vi "Ex 02 - Simple A-Scan (Low Level).vi"() -> ()   [LabVIEW 2026]
uses:
  <instrlib>/MicroPulse/Public/Data/Datatypes/TCP config.ctl
  <instrlib>/MicroPulse/Public/Data/Datatypes/MP - data output format.ctl
  <instrlib>/MicroPulse/Public/Data/Datatypes/MP - pulser voltage.ctl
  <instrlib>/MicroPulse/Public/Data/Datatypes/MP - pulse damping.ctl
  <instrlib>/MicroPulse/Public/Data/Datatypes/MP - frequency filter.ctl
  <instrlib>/MicroPulse/Public/Data/Datatypes/MP - waveform type.ctl
  <instrlib>/MicroPulse/Public/Data/Datatypes/MP - amplitude reporting mode.ctl
  <instrlib>/MicroPulse/Public/Data/Datatypes/MP - averaging.ctl
  <instrlib>/MicroPulse/Public/Data/Datatypes/MP - echo gate mode.ctl
  <instrlib>/MicroPulse/MicroPulse_Driver.lvlib
  <vilib>/ptbypt/NI_PtbyPt.lvlib
panel:
  out "Test No. Added":u32
  out "num messages":i32
  out "running average PRF":dbl format="%0.2f"
  out "error out":errorcluster
  out "System Messages":string
  out "Waveform Graph":u16[](graph)
  in  "stop":bool
  in  "TCP config":T1={"Connection ID"=refnum, "IP address"="10.1.1.2", "host port"=1067, "OC timeout"=5000, "Read timeout"=100, "Write timeout"=100} {"Write timeout" format="%dms"; "Read timeout" format="%dms"; "OC timeout" format="%dms"}
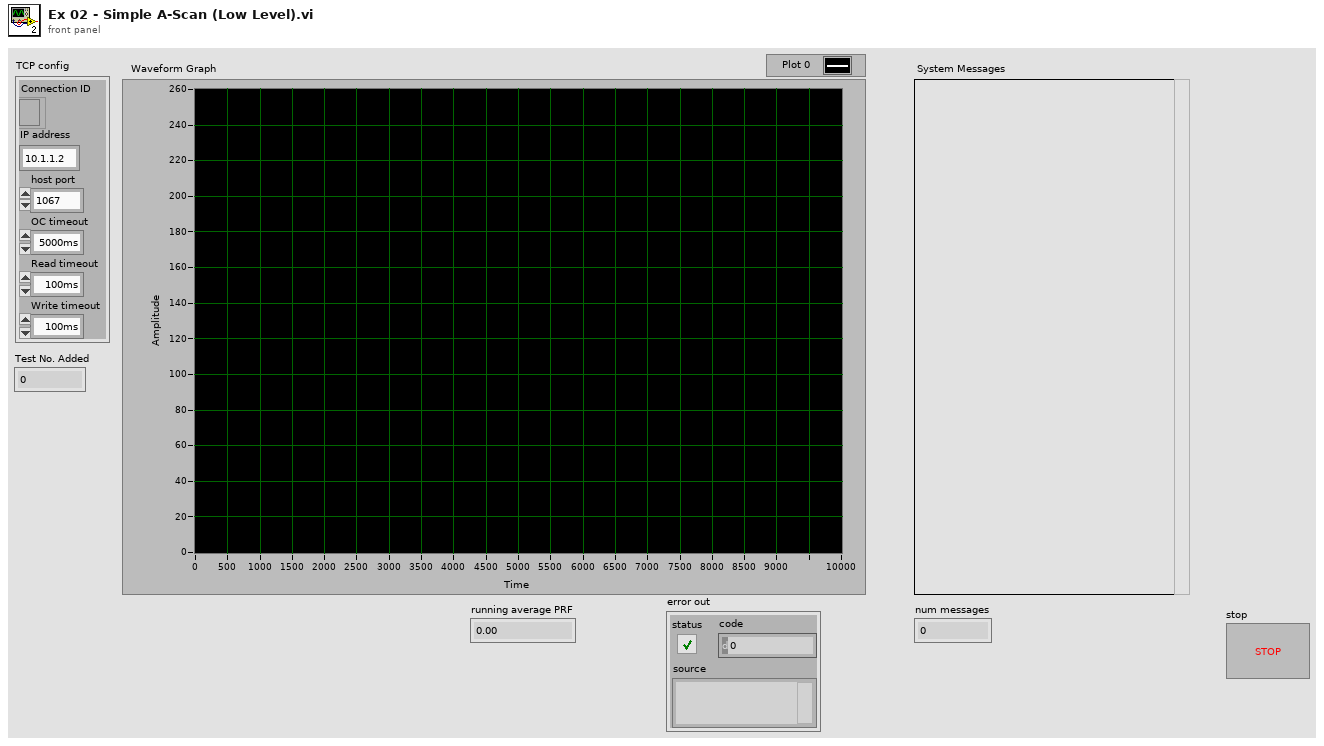
[diagram p1: front panel]
types:
  T1 = typedef "MicroPulse_Driver.lvlib/TCP config.ctl" = cluster{"Connection ID":refnum<k5>, "IP address":string, "host port":u16, "OC timeout":i32, "Read timeout":i32, "Write timeout":i32}
  T2 = typedef "MicroPulse_Driver.lvlib/MP - echo gate mode.ctl" = enum16{"Echo Trigger OFF", "Echo Gate Display Mode", "Echo Trigger ON", "Multi Gate or FMC Mode", "Reserved", "PA - Echo Trigger ON"}
  T3 = typedef "MicroPulse_Driver.lvlib/MP - averaging.ctl" = enum16{"None", "2", "4", "8", "16", "32", "64", "128", "256"}
  T4 = typedef "MicroPulse_Driver.lvlib/MP - amplitude reporting mode.ctl" = enum16{"1st Peak in gate", "Maximum Peak in gate", "All Peaks", "Ascan Data", "1st Threshold Crossing Peak", "Ascan + Peaks", "All Peaks for Multigate", "Peaks + Ascan for Multigate", "Peaks + P_Ascan for Multigate", "Full Matrix Capture"}
  T5 = typedef "MicroPulse_Driver.lvlib/MP - waveform type.ctl" = enum16{"Rectified Signal", "RF Signal", "+Half Wave", "-Half Wave"}
  T6 = typedef "MicroPulse_Driver.lvlib/MP - frequency filter.ctl" = enum16{"No change", "1MHz Bandpass", "2MHz Bandpass", "4MHz Bandpass", "5MHz Bandpass", "10MHz Bandpass", "2.5-18MHz Broadband", "0.75-12MHz  Broadband", "0.5MHz Bandpass", "5MHz 2nd Order TOFD", "10MHz 2nd Order TOFD", "3.0-25MHz Broadband", "3.0-30MHz Broadband"}
  T7 = typedef "MicroPulse_Driver.lvlib/MP - pulse damping.ctl" = enum16{"660W", "458W", "220W", "149W", "102W", "82W", "63W", "51W"}
  T8 = typedef "MicroPulse_Driver.lvlib/MP - pulser voltage.ctl" = enum16{"50V", "100V", "150V", "200V", "250V", "300V"}
  T9 = typedef "MicroPulse_Driver.lvlib/MP - data output format.ctl" = enum16{"", "8-bit Mode", "10-bit Mode", "12-bit Mode", "16-bit Mode", "8-bit Log Mode", "12-bit Packed Mode"}
  T10 = typedef "MicroPulse_Driver.lvlib/MP - scan data info.ctl" = cluster{"Message Header":u16, "Error Message":u16, "Test No.":u32, "Channel No.":u8, "Sweep No.":u32, "Gate No.":u32, "DOF":T9, "retain data":T11, "scan data":u16[], "scan length":i32, "scan index":i32, "peak data":cluster{"timebase":u16[], "data":u16[]}, "#peaks":i32, "PRF":dbl, "IP":cluster{"Axis No.":u8, "Location":u32, "MIP location":u32, "MIP?":bool}, "echo range":u16, "ETG":bool, "CAL 0 complete":bool, "Axis Positions":T12}
  T11 = typedef "MicroPulse_Driver.lvlib/MP - retain scan.ctl" = enum16{"None", "Ascan", "Peaks"}
  T12 = typedef "MicroPulse_Driver.lvlib/MP - axis positions (LLC).ctl" = cluster{"Axis 1":u32, "Axis 2":u32, "Axis 3":u32, "Axis 4":u32, "Status":u8}
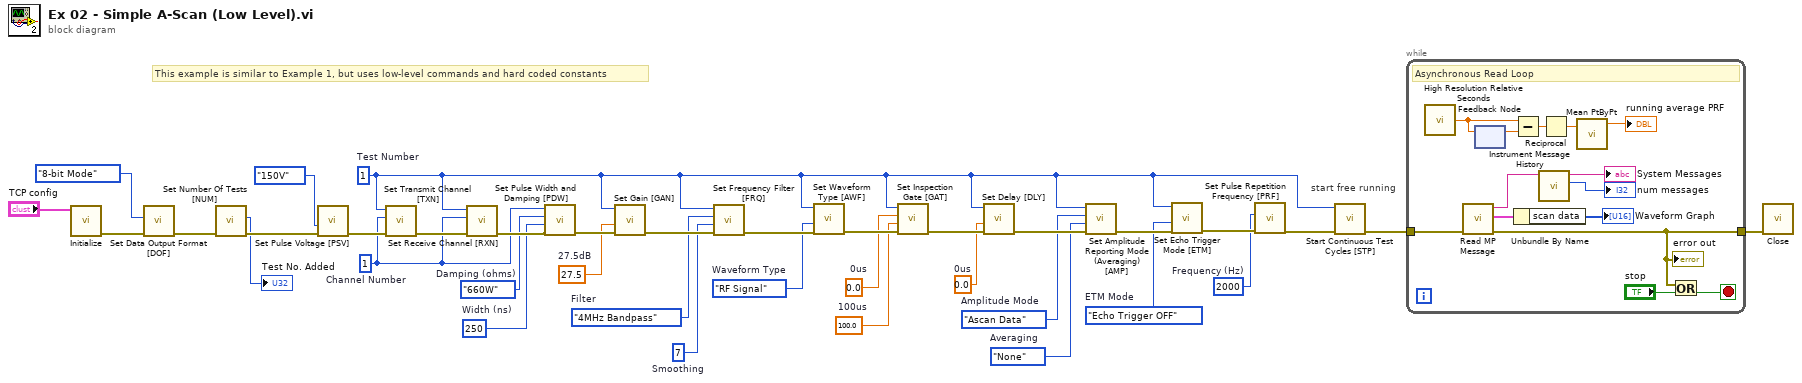
[diagram p0: block diagram]
diagram:
  w9 = u16 2000  # Frequency (Hz)
  w11 = MP_-_echo_gate_mode."Echo Trigger OFF"  # ETM Mode
  w13 = MP_-_averaging."None"  # Averaging
  w14 = MP_-_amplitude_reporting_mode."Ascan Data"  # Amplitude Mode
  w16 = 0.0  # 0us
  w18 = 100.0  # 100us
  w19 = 0.0  # 0us
  w21 = MP_-_waveform_type."RF Signal"  # Waveform Type
  w23 = u16 7  # Smoothing
  w24 = MP_-_frequency_filter."4MHz Bandpass"  # Filter
  w26 = 27.5  # 27.5dB
  w28 = u32 250  # Width (ns)
  w29 = MP_-_pulse_damping."660W"  # Damping (ohms)
  w30 = u32 1  # Channel Number
  w4 = u32 1  # Test Number
  # "This example is similar to Example 1, but uses low-level commands and hard coded constants"
  # "start free running"
  n1 = call <instrlib>:"Initialize.vi"("TCP config"="TCP config") -> ("error out"=w3:errorcluster)  [unwired: 9 in, 1 out]
  n2 = call "Set Data Output Format [DOF].vi"("error in (no error)"=w3, "Mode"=MP_-_data_output_format."8-bit Mode") -> ("error out"=w8:errorcluster)  [unwired: 8 in, 1 out]
  n3 = call <instrlib>:"Set Number Of Tests [NUM].vi"("error in (no error)"=w8) -> ("error out"=w7:errorcluster, "Test No. Added"=→"Test No. Added":u32)  [unwired: 8 in, 1 out]
  n4 = call <instrlib>:"Set Pulse Voltage [PSV].vi"("error in (no error)"=w7, "Voltage"=MP_-_pulser_voltage."150V") -> ("error out"=w33:errorcluster)  [unwired: 8 in, 1 out]
  n5 = call <instrlib>:"Set Transmit Channel [TXN].vi"("error in (no error)"=w33, "Channel Number"=w30, "Test Number"=w4) -> ("error out"=w32:errorcluster)  [unwired: 7 in, 1 out]
  n6 = call <instrlib>:"Set Receive Channel [RXN].vi"("error in (no error)"=w32, "Channel Number"=w30, "Test Number"=w4) -> ("error out"=w31:errorcluster)  [unwired: 7 in, 1 out]
  n7 = call <instrlib>:"Set Pulse Width and Damping [PDW].vi"("error in (no error)"=w31, "Width (ns)"=w28, "Damping"=w29, "Channel Number"=w30) -> ("error out"=w27:errorcluster)  [unwired: 6 in, 1 out]
  n8 = call <instrlib>:"Set Gain [GAN].vi"("error in (no error)"=w27, "Gain (dB)"=w26, "Test Number"=w4) -> ("error out"=w25:errorcluster)  [unwired: 7 in, 1 out]
  n9 = call <instrlib>:"Set Frequency Filter [FRQ].vi"("error in (no error)"=w25, "Smoothing"=w23, "Filter"=w24, "Test Number"=w4) -> ("error out"=w22:errorcluster)  [unwired: 6 in, 1 out]
  n10 = call <instrlib>:"Set Waveform Type [AWF].vi"("error in (no error)"=w22, "Waveform Type"=w21, "Test Number"=w4) -> ("error out"=w20:errorcluster)  [unwired: 7 in, 1 out]
  n11 = call <instrlib>:"Set Inspection Gate [GAT].vi"("error in (no error)"=w20, "Gate Length (us)"=w18, "Gate Start (us)"=w19, "Test Number"=w4) -> ("error out"=w17:errorcluster)  [unwired: 6 in, 1 out]
  n12 = call <instrlib>:"Set Delay [DLY].vi"("error in (no error)"=w17, "Delay (us)"=w16, "Test Number"=w4) -> ("error out"=w15:errorcluster)  [unwired: 7 in, 1 out]
  n13 = call <instrlib>:"Set Amplitude Reporting Mode (Averaging) [AMP].vi"("error in (no error)"=w15, "Averaging"=w13, "Amplitude Mode"=w14, "Test Number"=w4) -> ("error out"=w12:errorcluster)  [unwired: 6 in, 1 out]
  n14 = call <instrlib>:"Set Echo Trigger Mode [ETM].vi"("error in (no error)"=w12, "ETM Mode"=w11, "Test Number"=w4) -> ("error out"=w10:errorcluster)  [unwired: 7 in, 1 out]
  n15 = call <instrlib>:"Set Pulse Repetition Frequency [PRF].vi"("error in (no error)"=w10, "Frequency (Hz)"=w9) -> ("error out"=w6:errorcluster)  [unwired: 8 in, 1 out]
  n16 = call <instrlib>:"Start Continuous Test Cycles [STP].vi"("error in (no error)"=w6, "Test Number"=w4) -> ("error out"=w2:errorcluster)  [unwired: 8 in, 1 out]
  n17 = while {
    tunnel: [w38] -> w5
    tunnel: w2 -> [w37]
    stop <- w39 stop-if-true
    # "Asynchronous Read Loop"
    n18 = call <vilib>:"High Resolution Relative Seconds.vi"() -> ("relative seconds"=w47:dbl)
    n19 = call <instrlib>:"Read MP Message.vi"("error in (no error)"=w37) -> ("error out"=w38:errorcluster, "scan data info"=w49:T10, "Instrument Message"=w42:string)  [unwired: 6 in, 2 out]
    "error out" <- w38
    n20 = feedback-in #1(w47) -> ()
    n21 = feedback #1() -> (w46:dbl)  [unwired: 1 in]
    n22 = Subtract(x=w47, y=w46) -> (x-y=w45:dbl)
    n23 = Unbundle By Name(w49) -> ("scan data"=→"Waveform Graph":u16[])
    n24 = call <instrlib>:"Instrument Message History.vi"("Instrument Message"=w42) -> ("Message Count"=→"num messages":i32, "Message History out"=→"System Messages":string)  [unwired: 9 in]
    n25 = Reciprocal(x=w45) -> (1/x=w44:dbl)
    n26 = call <vilib>:"Mean PtByPt.vi"("x"=w44) -> ("mean"=→"running average PRF":dbl)  [unwired: 3 in, 1 out]
    n27 = Or(x=w38, y="stop") -> (x .or. y?=w39:bool)
  }
  n28 = call <instrlib>:"Close.vi"("error in (no error)"=w5) -> ()  [unwired: 9 in, 2 out]
